vi "DAQ_PW_Read_Vsource_Update_to_DEV_Global.vi"(11 "USB_DEV_1 in":string) -> (3 "USB_DEV_1 out":string)   [LabVIEW 2015]
uses:
  Share Data/uPower_kit.ctl
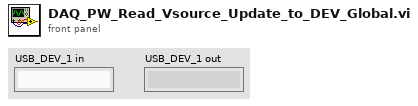
[diagram p1: front panel]
types:
  T1 = typedef "uPower_kit.ctl" = cluster{"DEV":string, "BUSY":bool, "VBAT":dbl, "OUTPUT":bool, "LAST_RESULT":dbl, "DURATION":u16, "TRIGGER":bool, "RANGE":string, "Vsource":dbl}
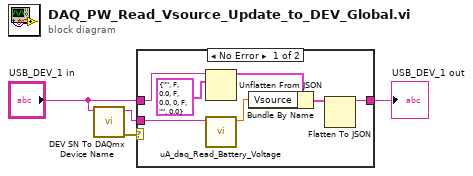
[diagram p0: block diagram]
diagram:
  n1 = call "DEV SN To DAQmx Device Name.vi"("USN_DEV (JSON)"="USB_DEV_1 in") -> ("error out"=w2:errorcluster, "DAQmx Device Name"=w1:tag)  [unwired: 9 in]
  n2 = case shown="No Error" w2 {
    tunnel: w1 -> [w11 _]
    tunnel: "USB_DEV_1 in" -> [w7 w12]
    tunnel: [w5 w12] -> w4
    frame No Error {
      n3 = Unflatten From JSON(JSON string=w7, type and defaults=T1 {"DEV"="", "BUSY"=FALSE, "VBAT"=0.0, "OUTPUT"=FALSE, "LAST_RESULT"=0.0, "DURATION"=0, "TRIGGER"=FALSE, "RANGE"="", "Vsource"=0.0} ("DEV_BUSY")) -> (value=w6:T1)  [unwired: 5 in, 1 out]
      n4 = call "uA_daq_Read_Battery_Voltage.vi"("USB DAQ"=w11) -> ("Battery_Voltage"=w8:dbl)  [unwired: 9 in, 1 out]
      n5 = Bundle By Name(cluster=w6, "Vsource"=w8) -> (w9:T1)
      n6 = Flatten To JSON(anything=w9) -> (JSON string=w5:string)  [unwired: 2 in, 1 out]
    }
    frame Error {
    }
  }
  "USB_DEV_1 out" <- w4
